vi "Configure Amplifier State.vi"(8 "error in (no error)":errorcluster, 10 "lamp enabled":bool, 11 "Lotis in":refnum<class "PL Lotis TII LS.lvclass">) -> (0 "error out":errorcluster, 3 "Lotis out":refnum<class "PL Lotis TII LS.lvclass">)   [LabVIEW 2015, in "PL Lotis TII LS.lvclass"]
doc: "Configures amplifier state."
uses:
  PL Lotis TII LS.lvclass
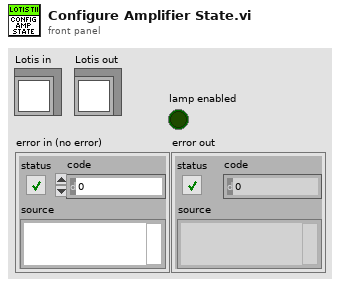
[diagram p1: front panel]
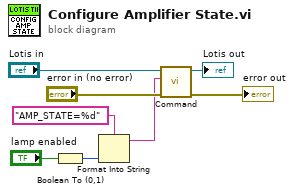
[diagram p0: block diagram]
diagram:
  n1 = Boolean To (0,1)(Boolean="lamp enabled") -> (0, 1=w1:i16)
  n2 = Format Into String(format string="AMP_STATE=%d" ("command"), w1) -> (resulting string=w3:string)  [unwired: 2 in, 1 out]
  n3 = call "Command.vi"("error in (no error)"="error in (no error)", "command"=w3, "Lotis in"="Lotis in") -> ("error out"=→"error out":errorcluster, "Lotis out"=→"Lotis out":refnum<class "PL Lotis TII LS.lvclass">)  [unwired: 6 in, 1 out]
